vi "OSM.vi"(0 "System no.":i32=1 min=1 max=4 step=1, 2 "Affected channels":string[](array[string]), 3 "No. of steps":dbl[](array[numeric]), 4 "No.of digits":i16, 5 "error in":errorcluster) -> (19 "error out":errorcluster)   [LabVIEW 2020]
doc: "Open loop step moving of given channels or axes. Use SSA.vi (if available) to set step size. \n\nC-891: Only valid for devices with stepper motors.\n\nE-135: The SSA command is not supported by the E-135. To change the step size, please use the SPA command to change the corresponding parameter (parameter ID 0x23000500).\n\nE-712: To change between nanostepping mode and full-step mode use parameter \"PiezoWalk Driving Mode\" (ID 0x07001a00, can be changed with SPA and SEP). The No. of steps to perform can always be given as floating-point number, but depending on the driving mode selection made with the PiezoWalk Driving Mode parameter, processing of the value differs:\nFull-step mode: decimal places are discarded. This means that only complete step cycles are performed. Set No. of digits to 0 for speed of transmission. \nNanostepping mode: floating-point numbers are processed. Make sure to increase No. of digits. This means that also parts of a complete step cycle are performed.\nPrior to using this command, servo must be disabled for the axis to which the PiezoWalk channel is assigned. \n\nE-755: No. of digits = 0\n\nE-861: The velocity for open-loop step motion depends on the step size and on the step frequency. The step size is given by the amplitude of the transport voltage which can be set with SSA and queried with SSA?. The step frequency can be set with OVL and queried with OVL?.\nIn open-loop operation, a RNP command must be sent each time the motion mode is to be changed from stepping motion (OSM command) to analog motion (OAD command) and vice versa. RNP brings the drive to a full-holding-force, zero-drive-voltage Relaxed state.\nThe first OSM sent for a NEXACT® linear drive which is in the Relaxed state prepares the drive for stepping motion (brings it to the In Motion state) before the actual motion is done. Once the drive is in the In Motion state, each subsequent OSM motion will be executed immediately.\nThe first OSM after a change of motion mode and the RNP procedure can take up to four times the slewrate value (parameter ID 0x7000002; can be changed with SPA and SEP).\nTo command parts of a step cycle, make sure to increase \"No. of digits\".\nMotion commands like OSM are not allowed when a joystick is active on the axis.\n\nE-870, E-872: The SSA command is not supported by the E-870 driver electronics. To change the step size, please use the SPA command to change the corresponding parameters.\n\nE-871, E-873:"
panel:
  # "Open loop step moving of given PiezoWalk channels. Use SSA.vi to \nset step size."
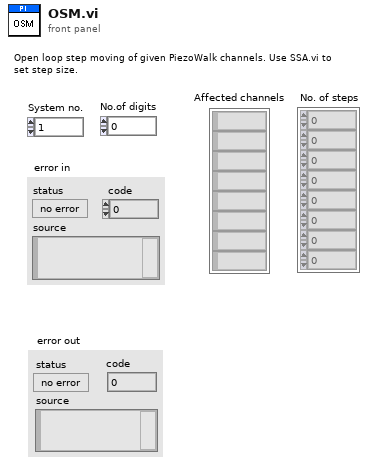
[diagram p1: front panel]
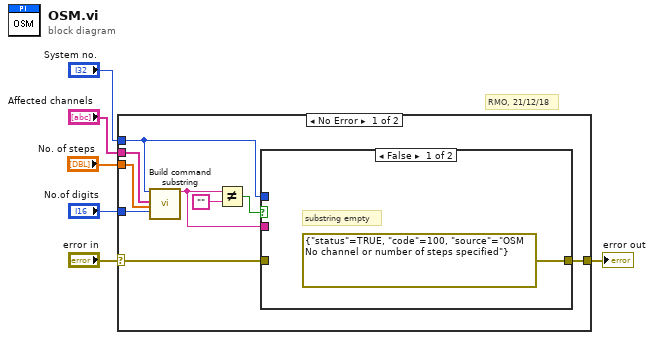
[diagram p0: block diagram]
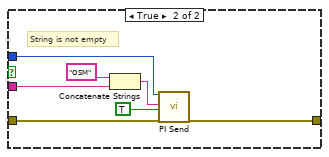
[diagram p2: hidden frame]
diagram:
  # "RMO, 21/12/18"
  n1 = case shown="No Error" "error in" {
    selector: "error in" -> [w7 w24]
    tunnel: [w15 w24] -> w6
    tunnel: "No. of steps" -> [w12 _]
    tunnel: "System no." -> [w9 _]
    tunnel: "Affected channels" -> [w11 _]
    tunnel: "No.of digits" -> [w8 _]
    frame No Error {
      n2 = call "Build command substring.vi"("System no."=w9, "Affected axes"=w11, "Parameters"=w12, "No. of digits"=w8) -> ("Command substring"=w13:string)  [unwired: 3 in, 12 out]
      n3 = Not Equal?(x=w13, y="") -> (x != y?=w10:bool)
      n4 = case shown="False" w10 {
        tunnel: w13 -> [_ w22]
        tunnel: [errorcluster {"status"=TRUE, "code"=100, "source"="OSM No channel or number of steps specified"} ("error out") w17] -> w15
        tunnel: w7 -> [_ w19]
        tunnel: w9 -> [_ w18]
        frame False {
          # "substring empty"
        }
        frame True {
          # "String is not empty"
          n5 = Concatenate Strings("OSM", w22) -> (w20:string)
          n6 = call "PI Send.vi"("System no."=w18, "String to send"=w20, "Attach termination char.?"=TRUE ("Attach Linefeed?"), "error in"=w19) -> ("error out"=w17:errorcluster)  [unwired: 2 in, 13 out]
        }
      }
    }
    frame Error {
    }
  }
  "error out" <- w6
